vi "FaultIndicator.vi"(11 "Fault in":bool) -> ()   [LabVIEW 2018]
uses:
  <vilib>/NI_Real-Time Target Support.lvlib
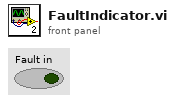
[diagram p1: front panel]
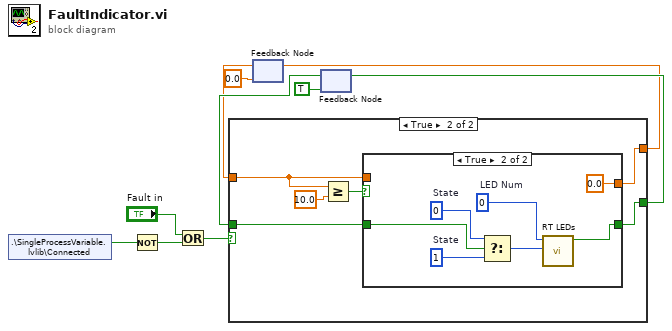
[diagram p0: block diagram]
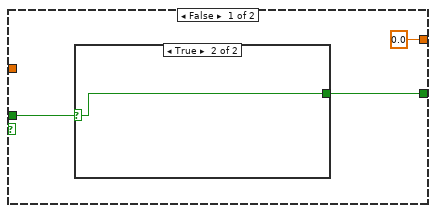
[diagram p2: hidden frame]
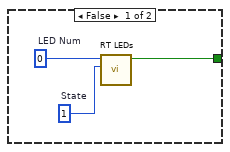
[diagram p3: hidden frame]
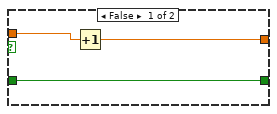
[diagram p4: hidden frame]
diagram:
  n1 = shared-variable ".\\SingleProcessVariable.lvlib\\Connected"() -> (w4:bool)  [unwired: 1 in, 1 out]
  n2 = Not(x=w4) -> (.not. x?=w3:bool)
  n3 = Or(x="Fault in", y=w3) -> (x .or. y?=w1:bool)
  n4 = feedback #1(0.0) -> (w7:dbl)
  n5 = feedback #2(TRUE ("Led State")) -> (w10:bool)
  n6 = case shown="True" w1 {
    tunnel: w10 -> [w13 w23]
    tunnel: [w12 w22] -> w9
    tunnel: w7 -> [_ w19]
    tunnel: [0.0 w18] -> w6
    frame False {
      n7 = case shown="True" w13 {
        selector: w13 -> [_ w17]
        tunnel: [w14 w17] -> w12
        frame False {
          w15 = 1  # State
          w16 = 0  # LED Num
          n8 = call <vilib>:"RT LEDs.vi"("State"=w15, "LED Num"=w16) -> ("Led State"=w14:bool)  [unwired: 4 in, 1 out]
        }
        frame True {
        }
      }
    }
    frame True {
      n9 = Greater Or Equal?(x=w19, y=10.0) -> (x >= y?=w21:bool)
      n10 = case shown="True" w21 {
        tunnel: w23 -> [w24 w31]
        tunnel: [w24 w28] -> w22
        tunnel: w19 -> [w26 _]
        tunnel: [w25 0.0] -> w18
        frame False {
          n11 = Increment(x=w26) -> (x+1=w25:dbl)
        }
        frame True {
          w30 = 0  # LED Num
          w32 = 1  # State
          w33 = 0  # State
          n12 = Select(t=w33, s=w31, f=w32) -> (s? t:f=w29:i32)
          n13 = call <vilib>:"RT LEDs.vi"("State"=w29, "LED Num"=w30) -> ("Led State"=w28:bool)  [unwired: 4 in, 1 out]
        }
      }
    }
  }
  n14 = feedback-in #1(w6) -> ()
  n15 = feedback-in #2(w9) -> ()
